vi "Call Command.vi"(11 "Command":T1={"Name"="", "CPTM.DataType"=variant, "All Control Values Variant"=[], "icon full"={"image type"=0, "image depth"=0, "image"=[], "mask"=[], "colors"=[], "Rectangle"={"left"=0, "top"=0, "right"=0, "bottom"=0}}, "icon scaled"={"image type"=0, "image depth"=0, "image"=[], "mask"=[], "colors"=[], "Rectangle"={"left"=0, "top"=0, "right"=0, "bottom"=0}}, "Path"=path "", "Subsystem Color"=16777216}) -> ()   [LabVIEW 2020]
uses:
  submodules/bordeaux-pathinator/Bordeaux/Types/Single Cmd Info.ctl
  <vilib>/picture/picture.llb/imagedata.ctl
panel:
  out "error out 2":errorcluster
  out "error out":errorcluster
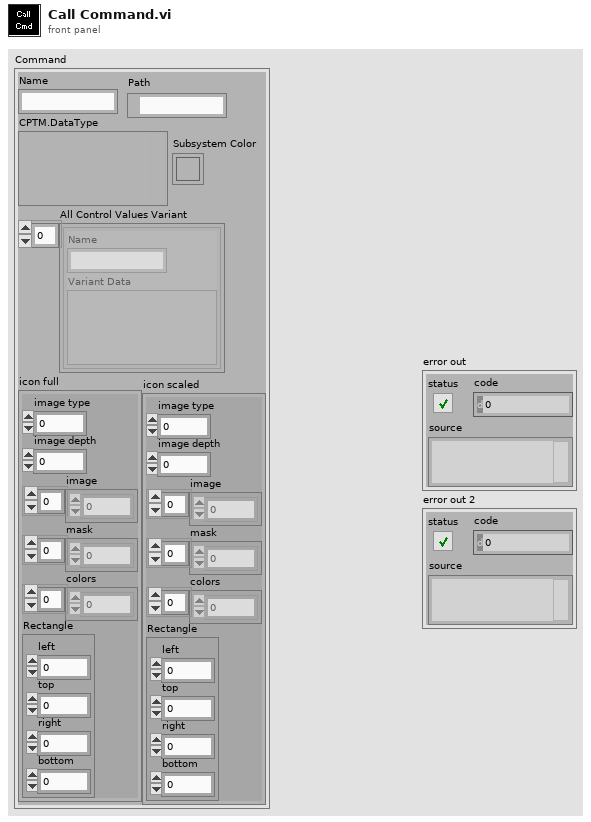
[diagram p1: front panel]
types:
  T1 = typedef "Single Cmd Info.ctl" = cluster{"Name":string, "CPTM.DataType":variant, "All Control Values Variant":cluster{"Name":string, "Variant Data":variant}[], "icon full":T2, "icon scaled":T2, "Path":path, "Subsystem Color":u32}
  T2 = typedef "imagedata.ctl" = cluster{"image type":i32, "image depth":i32, "image":u8[], "mask":u8[], "colors":u32[], "Rectangle":cluster{"left":i16, "top":i16, "right":i16, "bottom":i16}}
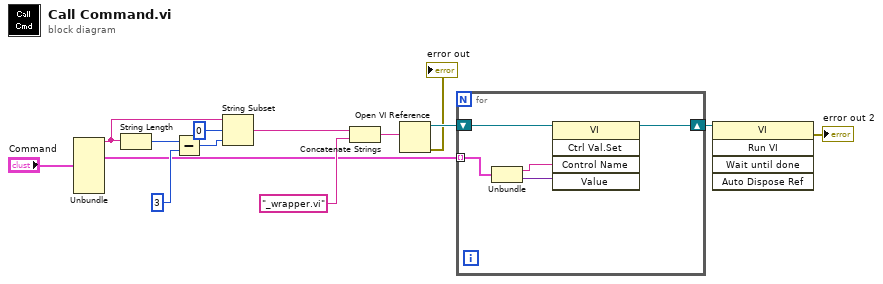
[diagram p0: block diagram]
diagram:
  n1 = Unbundle("Command") -> ("Name"=w4:string, "All Control Values Variant"=w8:cluster{"Name":string, "Variant Data":variant}[])  [unwired: 5 out]
  n2 = String Length(string=w4) -> (length=w13:i32)
  n3 = Subtract(x=w13, y=3) -> (x-y=w12:i32)
  n4 = String Subset(string=w4, offset (0)=0, length (rest)=w12) -> (substring=w10:string)
  n5 = Concatenate Strings(w10, "_wrapper.vi" ("string")) -> (w3:string)
  n6 = Open VI Reference(vi path=w3) -> (vi reference=w7:refnum<vi>, error out=→"error out":errorcluster)  [unwired: 5 in]
  n7 = for {
    tunnel: w8 -> [w17] mode=indexing
    shift-right: [w18] -> w6
    shift-left: w7 -> [w19]
    n8 = Unbundle(w17) -> ("Name"=w16:string, "Variant Data"=w15:variant)
    n9 = invoke class="VI" method="Ctrl Val.Set"(reference=w19, "Control Name"=w16, "Value"=w15) -> (reference out=w18:refnum<vi>)  [unwired: 2 in, 4 out]
  }
  n10 = invoke class="VI" method="Run VI"(reference=w6) -> (error out=→"error out 2":errorcluster)  [unwired: 4 in, 4 out]
